vi "AddDependency.vi"(8 "error in (no error)":errorcluster, 9 "Dependency":string, 11 "ProjectItem in":refnum<class "ProjectItem.lvclass">) -> (0 "error out":errorcluster, 3 "ProjectItem out":refnum<class "ProjectItem.lvclass">)   [LabVIEW 2019, in "SolutionBuilder.lvlib" / "ProjectItem.lvclass"]
uses:
  ProjectItem.lvclass
  ProjectItem.lvclass/ProjectItem.ctl
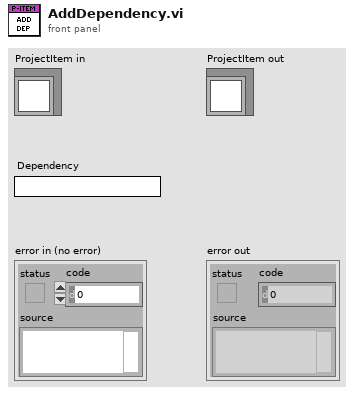
[diagram p1: front panel]
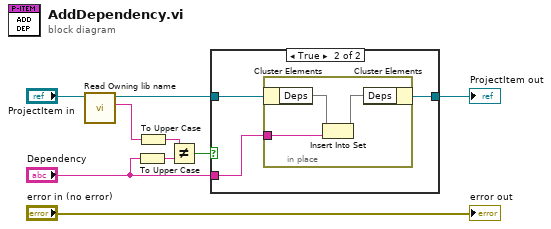
[diagram p0: block diagram]
diagram:
  n1 = call-dynamic "Read Owning lib name.vi"("ProjectItem in"="ProjectItem in") -> ("Owning lib name"=w1:string, "ProjectItem out"=w2:refnum<class "ProjectItem.lvclass">)  [unwired: 9 in]
  n2 = To Upper Case(1:"Dependency") -> (0:w6:string)
  n3 = To Upper Case(1:w1) -> (0:w7:string)
  n4 = Not Equal?(x=w7, y=w6) -> (x != y?=w4:bool)
  n5 = case shown="True" w4 {
    tunnel: [w10 w13] -> w8
    tunnel: w2 -> [w10 w12]
    tunnel: "Dependency" -> [_ w11]
    frame False {
    }
    frame True {
      n6 = in-place {
        in-place-border: w11 -> [w15]
        n7 = in-place-cluster #1(w12) -> ("Deps"=w16:set{string})
        n8 = Insert Into Set(10:w15, 11:w16) -> (3:w14:set{string})  [unwired: 1 out]
        n9 = in-place-cluster #1("Deps"=w14) -> (w13:refnum<class "ProjectItem.lvclass">)
      }
    }
  }
  "ProjectItem out" <- w8
  "error out" <- "error in (no error)"
